vi "tsa_AR Burg.vi"(9 "method":enum16{"Burg", "GL"}(ring), 10 "AR order":i32, 11 "response signal":dbl[](array[numeric]) format="%.2f") -> (0 "error":i32, 1 "noise variance":dbl format="%.2f", 2 "noise":dbl[](array[numeric]) format="%.2f", 3 "AR coefficents":dbl[](array[numeric]) format="%.2f", 4 "sita^2":dbl)   [LabVIEW 2010, in "NI_AALPro.lvlib"]
uses:
  NI_AALPro.lvlib
  Real Dot Product.vi
  NI_AALBase.lvlib
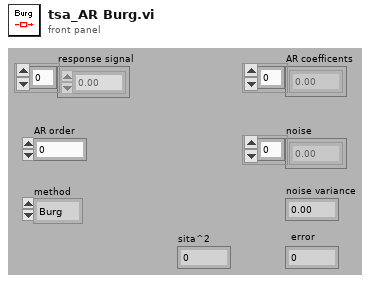
[diagram p1: front panel]
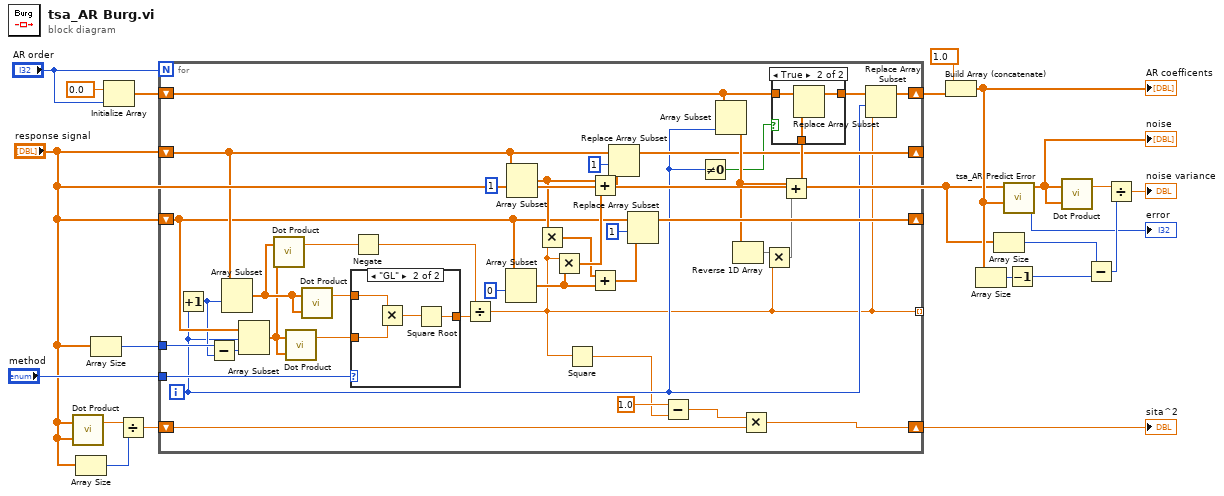
[diagram p0: block diagram]
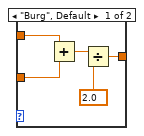
[diagram p3: hidden frame]
diagram:
  n1 = call-poly "Dot Product.vi"("Y Vector"="response signal", "X Vector"="response signal") -> ("X * Y"=w5:dbl)  [unwired: 1 out]
  n2 = Array Size(array="response signal") -> (size(s)=w2:i32)
  n3 = Array Size(array="response signal") -> (size(s)=w18:i32)
  n4 = Initialize Array(0.0 ("element"), "AR order") -> (w15:dbl[])
  n5 = Divide(x=w5, y=w2) -> (x/y=w4:dbl)
  n6 = for {
    N: "AR order" -> [_]
    shift-right: [w36] -> _
    shift-left: "response signal" -> [w53]
    shift-right: [w44] -> _
    shift-left: "response signal" -> [w47]
    tunnel: "method" -> [w61]
    shift-right: [w39] -> w17
    shift-left: w15 -> [w35]
    tunnel: w18 -> [w33]
    tunnel: [w27] -> _ mode=indexing
    shift-right: [w23] -> w1
    shift-left: w4 -> [w22]
    i -> [w29]
    n7 = Increment(x=w29) -> (x+1=w32:i32)
    n8 = Subtract(x=w33, y=w32) -> (x-y=w34:i32)
    n9 = Array Subset(array=w53, index=w32) -> (w58:dbl[])  [unwired: 1 in]
    n10 = Array Subset(array=w47, index=w29, length=w34) -> (w57:dbl[])
    n11 = call-poly "Dot Product.vi"("Y Vector"=w57, "X Vector"=w58) -> ("X * Y"=w56:dbl)  [unwired: 1 out]
    n12 = call-poly "Dot Product.vi"("Y Vector"=w57, "X Vector"=w57) -> ("X * Y"=w59:dbl)  [unwired: 1 out]
    n13 = call-poly "Dot Product.vi"("Y Vector"=w58, "X Vector"=w58) -> ("X * Y"=w60:dbl)  [unwired: 1 out]
    n14 = case shown="\"GL\"" w61 {
      tunnel: w60 -> [w70 w74]
      tunnel: w59 -> [w69 w73]
      tunnel: [w66 w71] -> w55
      frame "Burg", Default {
        n15 = Add(x=w70, y=w69) -> (x+y=w68:dbl)
        n16 = Divide(x=w68, y=2.0) -> (x/y=w66:dbl)
      }
      frame "GL" {
        n17 = Multiply(x=w74, y=w73) -> (x*y=w72:dbl)
        n18 = Square Root(x=w72) -> (sqrt(x)=w71:dbl)
      }
    }
    n19 = Negate(x=w56) -> (-x=w31:dbl)
    n20 = Divide(x=w31, y=w55) -> (x/y=w27:dbl)
    n21 = Array Subset(array=w47, index=0) -> (w28:dbl[])  [unwired: 1 in]
    n22 = Array Subset(array=w53, index=1) -> (w48:dbl[])  [unwired: 1 in]
    n23 = Multiply(x=w48, y=w27) -> (x*y=w43:dbl[])
    n24 = Multiply(x=w27, y=w28) -> (x*y=w50:dbl[])
    n25 = Square(x=w27) -> (x^2=w24:dbl)
    n26 = Add(x=w48, y=w50) -> (x+y=w49:dbl[])
    n27 = Add(x=w43, y=w28) -> (x+y=w45:dbl[])
    n28 = Replace Array Subset(array=w53, new element=w49, index=1) -> (w36:dbl[])
    n29 = Replace Array Subset(array=w47, new element=w45, index=1) -> (w44:dbl[])
    n30 = Subtract(x=1.0, y=w24) -> (x-y=w26:dbl)
    n31 = Not Equal To 0?(x=w29) -> (x != 0?=w30:bool)
    n32 = Array Subset(array=w35, length=w29) -> (w42:dbl[])  [unwired: 1 in]
    n33 = Reverse 1D Array(array=w42) -> (reversed array=w41:dbl[])
    n34 = Multiply(x=w26, y=w22) -> (x*y=w23:dbl)
    n35 = Multiply(x=w41, y=w27) -> (x*y=w40:dbl[])
    n36 = Add(x=w42, y=w40) -> (x+y=w37:dbl[])
    n37 = case shown="True" w30 {
      tunnel: [w62 w65] -> w38
      tunnel: w37 -> [_ w64]
      tunnel: w35 -> [w62 w63]
      frame False {
      }
      frame True {
        n38 = Replace Array Subset(array=w63, new element=w64) -> (w65:dbl[])  [unwired: 1 in]
      }
    }
    n39 = Replace Array Subset(array=w38, new element=w27, index=w29) -> (w39:dbl[])
  }
  "sita^2" <- w1
  n40 = Build Array (concatenate)(1.0, w17) -> (w11:dbl[])
  "AR coefficents" <- w11
  n41 = Array Size(array=w11) -> (size(s)=w10:i32)
  n42 = Array Size(array="response signal") -> (size(s)=w13:i32)
  n43 = call "tsa_AR Predict Error.vi"("Xt"="response signal", "AR coefficents"=w11) -> (7:"error"=w6:dbl[], 10:"error"=→"error":i32)  [unwired: 7 in]
  "noise" <- w6
  n44 = Decrement(x=w10) -> (x-1=w9:i32)
  n45 = call-poly "Dot Product.vi"("Y Vector"=w6, "X Vector"=w6) -> ("X * Y"=w14:dbl)  [unwired: 1 out]
  n46 = Subtract(x=w13, y=w9) -> (x-y=w12:i32)
  n47 = Divide(x=w14, y=w12) -> (x/y=→"noise variance":dbl)
